vi "Run Bfr Rx - Handle Rollover.vi"(7 "Offset in":u64, 8 "error in (no error)":errorcluster, 10 "Data in":u8[](array[numeric]), 11 "Buffer Size":i32) -> (0 "error out":errorcluster, 5 "Offset out":u64)   [LabVIEW 2016, in "UDP-Custom-Device Engine.lvlib"]
uses:
  UDP-Custom-Device Engine.lvlib
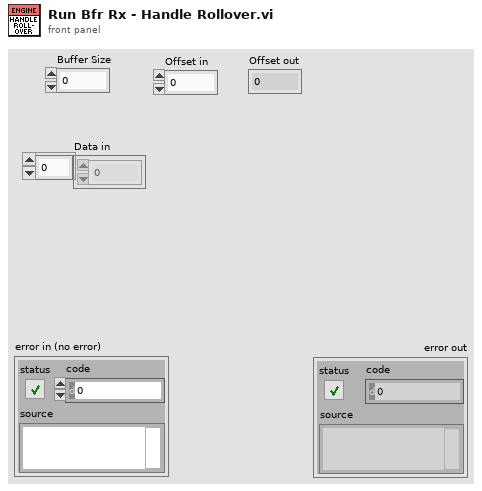
[diagram p1: front panel]
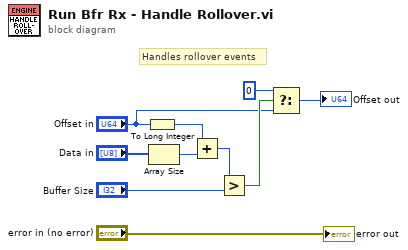
[diagram p0: block diagram]
diagram:
  # "Handles rollover events"
  n1 = To Long Integer(number="Offset in") -> (32bit integer=w9:i32)
  n2 = Array Size(array="Data in") -> (size(s)=w8:i32)
  n3 = Add(x=w9, y=w8) -> (x+y=w7:i32)
  n4 = Greater?(x=w7, y="Buffer Size") -> (0:w5:bool)
  n5 = Select(t=u64 0, s=w5, f="Offset in") -> (s? t:f=→"Offset out":u64)
  "error out" <- "error in (no error)"
